vi "StopSignal-WaitForComplete.vi"(8 "error in":errorcluster, 9 "timeout(ms)":i32=5000, 11 "StopSignal":T1) -> (0 "error out":errorcluster, 3 "StopSignal(dup)":T1)   [LabVIEW 2017, in "StopSignal.lvlib"]
uses:
  StopSignal.lvlib
  Typedef/StopSignal.ctl
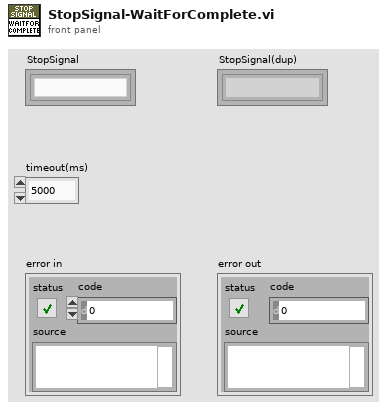
[diagram p1: front panel]
types:
  T1 = typedef "StopSignal.lvlib/StopSignal.ctl" = refnum<k1>
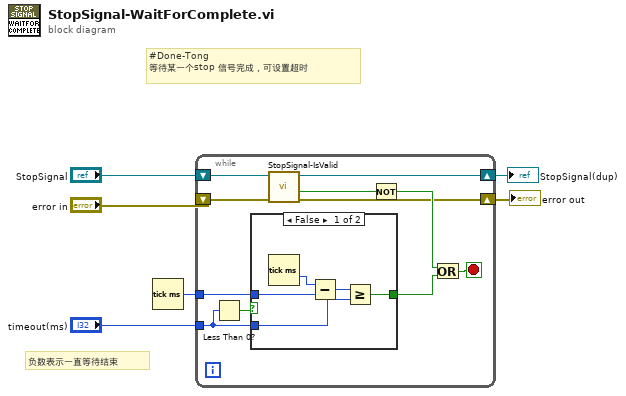
[diagram p0: block diagram]
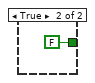
[diagram p2: hidden frame]
diagram:
  # "负数表示一直等待结束"
  # "#Done-Tong\n等待某一个stop 信号完成，可设置超时"
  n1 = Tick Count (ms)() -> (millisecond timer value=w5:u32)
  n2 = while {
    tunnel: w5 -> [w15]
    tunnel: "timeout(ms)" -> [w7]
    shift-right: [w11] -> w2
    shift-left: "error in" -> [w10]
    shift-right: [w9] -> w3
    shift-left: "StopSignal" -> [w16]
    stop <- w12 stop-if-true
    n3 = Less Than 0?(x=w7) -> (x < 0?=w8:bool)
    n4 = case shown="False" w8 {
      tunnel: w15 -> [w21 _]
      tunnel: w7 -> [w19 _]
      tunnel: [w18 FALSE] -> w13
      frame False {
        n5 = Tick Count (ms)() -> (millisecond timer value=w22:u32)
        n6 = Subtract(x=w22, y=w21) -> (x-y=w20:u32)
        n7 = Greater Or Equal?(x=w20, y=w19) -> (x >= y?=w18:bool)
      }
      frame True {
      }
    }
    n8 = call "StopSignal-IsValid.vi"("error in (no error)"=w10, "StopSignal"=w16) -> ("error out"=w11:errorcluster, "valid?"=w17:bool, "StopSignal(dup)"=w9:T1)  [unwired: 7 in]
    n9 = Not(x=w17) -> (.not. x?=w14:bool)
    n10 = Or(x=w14, y=w13) -> (x .or. y?=w12:bool)
  }
  "StopSignal(dup)" <- w3
  "error out" <- w2
